vi "Actor Core.vi"(8 "error in":errorcluster, 11 "Application in":refnum<class "Application.lvclass">) -> (0 "error out":errorcluster, 3 "Actor out":refnum<class "Actor.lvclass">)   [LabVIEW 2018, in "Application.lvlib" / "Application.lvclass"]
doc: "(<B>Filename</B>: Actor Framework.lvlib:Actor.lvclass:Actor Core.vi)\n\nReceives messages to the actor, reacts to them, and initiates any error handling that may shut the actor down.\n\nDescendant classes may override this VI to append parallel tasks for the actor to complete while it handles messages. Overrides use the Call Parent Method node."
uses:
  Application.lvclass
  C:/Program Files/National Instruments/LabVIEW 2018/vi.lib/ActorFramework/Actor/Actor.lvclass
  <vilib>/ActorFramework/Actor/Actor.lvclass
  Mode.ctl
  Resources/Type Defs/Camera Settings.ctl
  Application.lvclass/Application.ctl
  <vilib>/ActorFramework/Actor/Actor.lvclass/Actor.ctl
  <vilib>/ActorFramework/Message Enqueuer/Message Enqueuer.lvclass/Message Enqueuer.ctl
  Application Messages/Set All Laser Powers Msg/Set All Laser Powers Msg.lvclass/Set All Laser Powers Msg.ctl
  Application Messages/Start Autofocus Msg/Start Autofocus Msg.lvclass/Start Autofocus Msg.ctl
  Application Messages/Reset Laser Power Msg/Reset Laser Power Msg.lvclass/Reset Laser Power Msg.ctl
  Application Messages/Start Stream Msg/Start Stream Msg.lvclass/Start Stream Msg.ctl
  <vilib>/ActorFramework/Message Enqueuer/Init from Existing Queue.vi
  <vilib>/ActorFramework/Message Enqueuer/Enqueue.vi
  Application Messages/Stage Forward Msg/Stage Forward Msg.lvclass
  C:/Program Files/National Instruments/LabVIEW 2018/vi.lib/ActorFramework/Message/Message.lvclass
  Application Messages/Set All Laser Powers Msg/Set All Laser Powers Msg.lvclass
  Application Messages/Start Autofocus Msg/Start Autofocus Msg.lvclass
  Application Messages/Reset Laser Power Msg/Reset Laser Power Msg.lvclass
  Application Messages/Start Stream Msg/Start Stream Msg.lvclass
  <vilib>/ActorFramework/Message Priority Queue/Priority Enqueue.vi
  Wait for mode change.vi
  <vilib>/ActorFramework/Message Enqueuer/Message Enqueuer.lvclass
panel:
  in  "STOP":bool
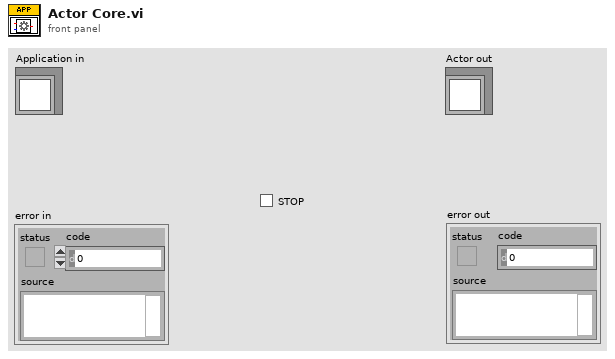
[diagram p1: front panel]
types:
  T1 = typedef "Camera Settings.ctl" = cluster{"Exposure Time (ms)":dbl, "Binning":enum16{"1x1", "2x2", "4x4"}, "Scan Mode":i32, "Frames to Acquire":dbl, "Pixel Correction":bool, "Frames to Skip":u32, "File Path":path, "Duty cycle":dbl, "ALEX":bool, "Shutter Enable":bool[], "Timelapse Interval (s)":u32}
  T2 = cluster{"Camera Settings":T1, "Auto-Advance":bool, "Auto Focus":bool, "Injection Countdown":bool, "Movies to acquire":i32}
  T3 = typedef "Mode.ctl" = enum16{"Idle", "Cancel", "Live", "Stream", "Autofocus", "Z-Stack"}
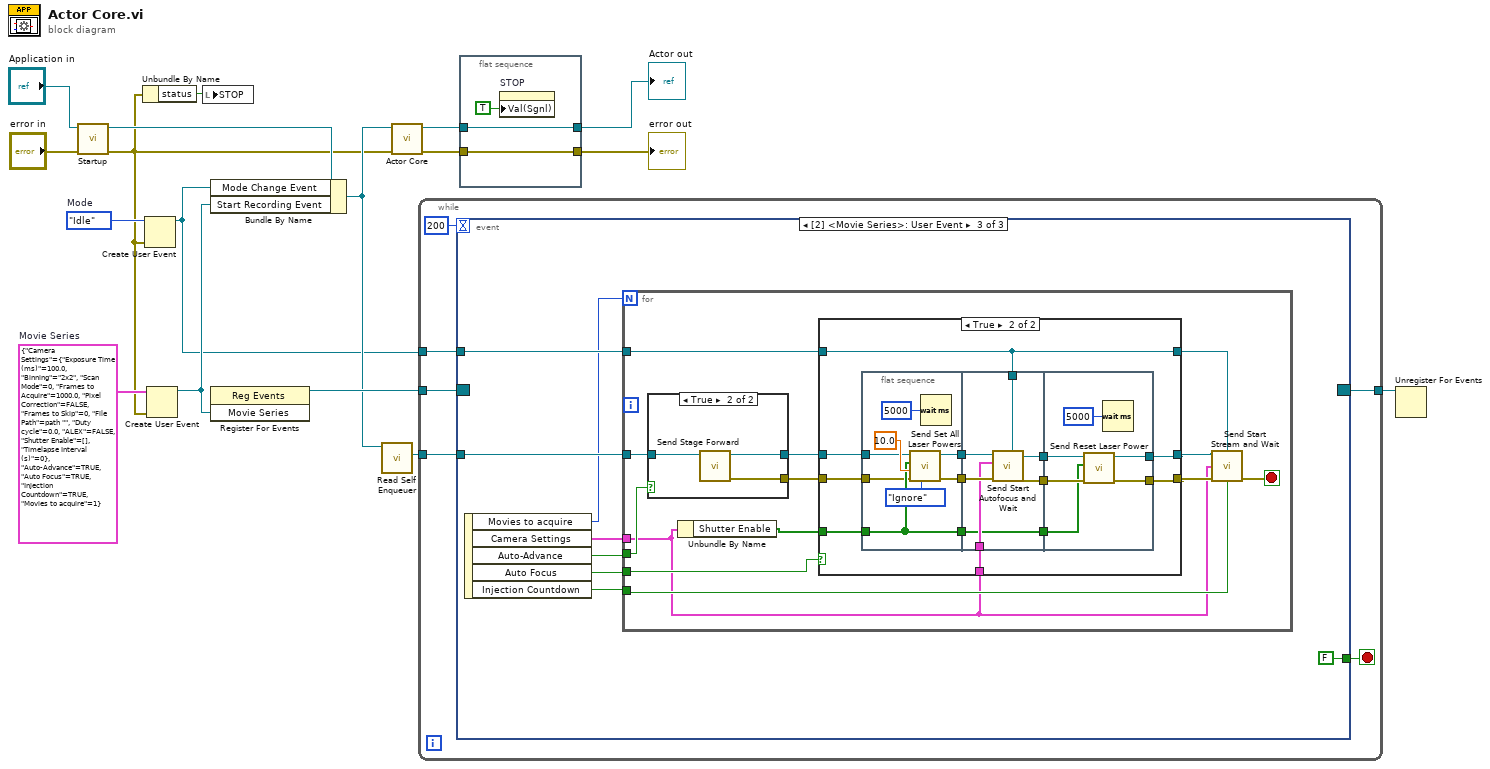
[diagram p0: block diagram]
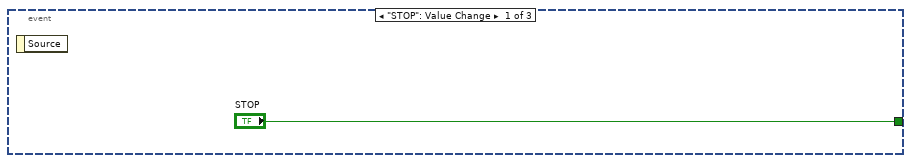
[diagram p2: hidden frame]
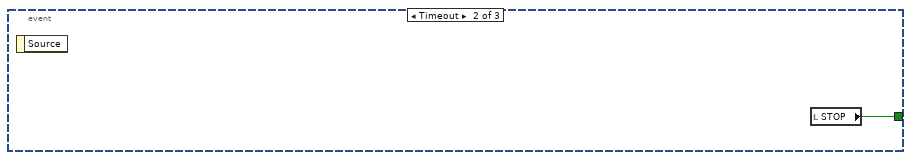
[diagram p3: hidden frame]
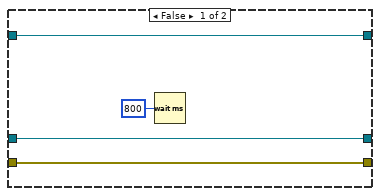
[diagram p4: hidden frame]
diagram:
  w13 = T2 {"Camera Settings"={"Exposure Time (ms)"=100.0, "Binning"=enum."2x2", "Scan Mode"=0, "Frames to Acquire"=1000.0, "Pixel Correction"=FALSE, "Frames to Skip"=0, "File Path"=path "", "Duty cycle"=0.0, "ALEX"=FALSE, "Shutter Enable"=[], "Timelapse Interval (s)"=0}, "Auto-Advance"=TRUE, "Auto Focus"=TRUE, "Injection Countdown"=TRUE, "Movies to acquire"=1}  # Movie Series
  w15 = Mode."Idle"  # Mode
  n1 = call-dynamic "Startup.vi"("error in (no error)"="error in", "Application in"="Application in") -> ("error out"=w2:errorcluster, "Application out"=w16:refnum<class "Application.lvclass">)  [unwired: 8 in]
  n2 = Unbundle By Name(w2) -> ("status"=w1:bool)
  n3 = Create User Event(user event datatype=w15, error in=w2) -> (user event=w3:refnum<user-event>)  [unwired: 1 out]
  n4 = Create User Event(user event datatype=w13, error in=w2) -> (user event=w10:refnum<user-event>)  [unwired: 1 out]
  n5 = local write "STOP"(w1) -> ()
  n6 = Bundle By Name(cluster=w16, "Mode Change Event"=w3, "Start Recording Event"=w10) -> (w12:refnum<class "Application.lvclass">)
  n7 = register-events(w10) -> (reference out=w14:refnum<event-registration>)  [unwired: 2 in, 1 out]
  n8 = call <vilib>:"Read Self Enqueuer.vi"("Actor"=w12) -> ("Self Enqueuer"=w11:refnum<class "Message Enqueuer.lvclass">)  [unwired: 10 in]
  n9 = call-parent "Actor Core.vi"("error in"=w2, "Actor in"=w12) -> ("error out"=w9:errorcluster, "Actor out"=w7:refnum<class "Actor.lvclass">)  [unwired: 8 in]
  n10 = while {
    tunnel: w14 -> [w23]
    tunnel: w11 -> [w21]
    tunnel: [w20] -> w4
    tunnel: w3 -> [w19]
    stop <- w22 stop-if-true
    n11 = event shown="[2] <Movie Series>: User Event" {
      selector: w23 -> [_ _ _]
      dyn-events: [_ _ _] -> w20
      timeout: 200 -> [_ _ _]
      tunnel: ["STOP" w25 FALSE ("STOP")] -> w22
      tunnel: w21 -> [_ _ w32]
      tunnel: w19 -> [_ _ w30]
      event "STOP": Value Change {
        n12 = event-data() -> ()  [unwired: 1 in, 1 out]
      }
      event Timeout {
        n13 = event-data() -> ()  [unwired: 1 in, 1 out]
        n14 = local read "STOP"() -> (w25:bool)
      }
      event User Event {
        n15 = event-data() -> ("Movies to acquire"=w26:i32, "Camera Settings"=w28:T1, "Auto-Advance"=w33:bool, "Auto Focus"=w31:bool, "Injection Countdown"=w27:bool)  [unwired: 1 in]
        n16 = for {
          N: w26 -> [_]
          tunnel: w33 -> [w45]
          tunnel: w32 -> [w44]
          tunnel: w31 -> [w42]
          tunnel: w30 -> [w41]
          tunnel: w28 -> [w35]
          tunnel: w27 -> [w37]
          stop <- w36 stop-if-true
          n17 = case shown="True" w45 {
            tunnel: [_ w88] -> w46
            tunnel: w44 -> [w85 w87]
            tunnel: [w85 w86] -> w43
            frame False {
            }
            frame True {
              n18 = call "Send Stage Forward.vi"("Message Enqueuer"=w87) -> ("error out"=w88:errorcluster, "Message Enqueuer out"=w86:refnum<class "Message Enqueuer.lvclass">)  [unwired: 9 in]
            }
          }
          n19 = Unbundle By Name(w35) -> ("Shutter Enable"=w34:bool[])
          n20 = case shown="True" w42 {
            tunnel: w46 -> [w49 w51]
            tunnel: [w49 w57] -> w39
            tunnel: w35 -> [_ w59]
            tunnel: w43 -> [w50 w62]
            tunnel: [w50 w56] -> w40
            tunnel: w41 -> [w48 w58]
            tunnel: [w48 w58] -> w38
            tunnel: w34 -> [_ w63]
            frame False {
              n21 = Wait (ms)(milliseconds to wait=u32 800) -> ()  [unwired: 1 out]
            }
            frame True {
              n22 = flat-sequence {
                tunnel: w63 -> [w66]
                tunnel: w62 -> [w68]
                tunnel: [w70] -> w61
                tunnel: [w67] -> w60
                tunnel: [w66] -> w52
                tunnel: w51 -> [w65]
                tunnel: w61 -> [w77]
                tunnel: w60 -> [w78]
                tunnel: w59 -> [w76]
                tunnel: w58 -> [w75]
                tunnel: [w74] -> w55
                tunnel: [w73] -> w54
                tunnel: [w72] -> w53
                tunnel: w52 -> [w72]
                tunnel: [w84] -> w57
                tunnel: [w83] -> w56
                tunnel: w55 -> [w82]
                tunnel: w54 -> [w81]
                tunnel: w53 -> [w80]
                frame #0 {
                  n23 = call "Send Set All Laser Powers.vi"("Mode"=enum16{"Normal", "Ignore", "Reset"}."Ignore", "error in (no error)"=w65, "Power"=10.0, "Line Enable"=w66, "Message Enqueuer"=w68) -> ("error out"=w70:errorcluster, "Message Enqueuer out"=w67:refnum<class "Message Enqueuer.lvclass">)  [unwired: 5 in]
                  n24 = Wait (ms)(milliseconds to wait=u32 5000) -> ()  [unwired: 1 out]
                }
                frame #1 {
                  n25 = call "Send Start Autofocus and Wait.vi"("Mode"=w75, "error in (no error)"=w77, "Camera Settings"=w76, "Message Enqueuer"=w78) -> ("error out"=w73:errorcluster, "Message Enqueuer out"=w74:refnum<class "Message Enqueuer.lvclass">)  [unwired: 6 in]
                }
                frame #2 {
                  n26 = call "Send Reset Laser Power.vi"("error in (no error)"=w81, "Shutter Enable"=w80, "Message Enqueuer"=w82) -> ("error out"=w84:errorcluster, "Message Enqueuer out"=w83:refnum<class "Message Enqueuer.lvclass">)  [unwired: 7 in]
                  n27 = Wait (ms)(milliseconds to wait=u32 5000) -> ()  [unwired: 1 out]
                }
              }
            }
          }
          n28 = call "Send Start Stream and Wait.vi"("Message Enqueuer"=w40, "Mode"=w38, "Camera Settings"=w35, "error in (no error)"=w39, "Injection Countdown"=w37) -> ("error out"=w36:errorcluster)  [unwired: 9 in, 1 out]
        }
      }
    }
  }
  n29 = flat-sequence {
    tunnel: w9 -> [w90]
    tunnel: [w90] -> w8
    tunnel: w7 -> [w89]
    tunnel: [w89] -> w6
    frame #0 {
      n30 = property on="STOP" class="Bool (strict)"("Val(Sgnl)"=TRUE) -> ()  [unwired: 2 in, 2 out]
    }
  }
  n31 = Unregister For Events(event registration refnum=w4) -> ()  [unwired: 1 in, 1 out]
  "error out" <- w8
  "Actor out" <- w6
